vi "preview date info.vi"(6 "DateTimeOrginal":timestamp, 8 "error in":errorcluster, 11 "Cluster in":T1={"Running VI"=refnum, "Test VI"=refnum, "Q Ref"=refnum, "UE"=refnum, "Data"=variant, "Timeout"=-1, "ListBox[]"=[], "Source Path"=path "", "Delta Time"=0.0, "ExifInfo[]"=[], "ListIndex"=0, "counter"=0, "Format"=enum."Files Only", "total"=0, "Operation"=enum."Read Info", "Status"=""} {"ExifInfo[]"."New DateTime" format="%<%.3X>T"; "ExifInfo[]"."DateTimeOrginal" format="%<%.3X>T"}) -> (0 "error out":errorcluster, 3 "Cluster out":T1={"Running VI"=refnum, "Test VI"=refnum, "Q Ref"=refnum, "UE"=refnum, "Data"=variant, "Timeout"=-1, "ListBox[]"=[], "Source Path"=path "", "Delta Time"=0.0, "ExifInfo[]"=[], "ListIndex"=0, "counter"=0, "Format"=enum."Files Only", "total"=0, "Operation"=enum."Read Info", "Status"=""} {"ExifInfo[]"."New DateTime" format="%<%.3X>T"; "ExifInfo[]"."DateTimeOrginal" format="%<%.3X>T"})   [LabVIEW 2023, in "EXIF Modifier.lvlib"]
uses:
  Controls/exif_consumer cluster.ctl
  Controls/exif_info cluster.ctl
  EXIF Modifier.lvlib
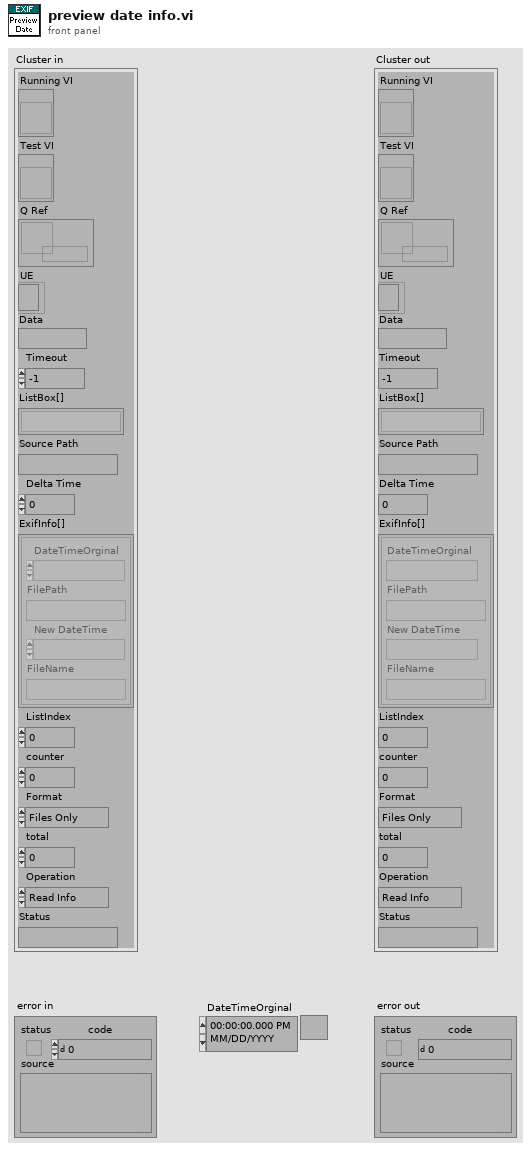
[diagram p1: front panel]
types:
  T1 = typedef "EXIF Modifier.lvlib/exif_consumer cluster.ctl" = cluster{"Running VI":refnum<vi>, "Test VI":refnum<vi>, "Q Ref":refnum<queue>, "UE":refnum<event-registration>, "Data":variant, "Timeout":i32, "ListBox[]":string[][], "Source Path":path, "Delta Time":dbl, "ExifInfo[]":T2[], "ListIndex":i32, "counter":i32, "Format":enum16{"Files Only", "Files Date", "All"}, "total":i32, "Operation":enum16{"Read Info", "Write Info"}, "Status":string}
  T2 = typedef "EXIF Modifier.lvlib/exif_info cluster.ctl" = cluster{"DateTimeOrginal":timestamp, "FilePath":path, "New DateTime":timestamp, "FileName":string}
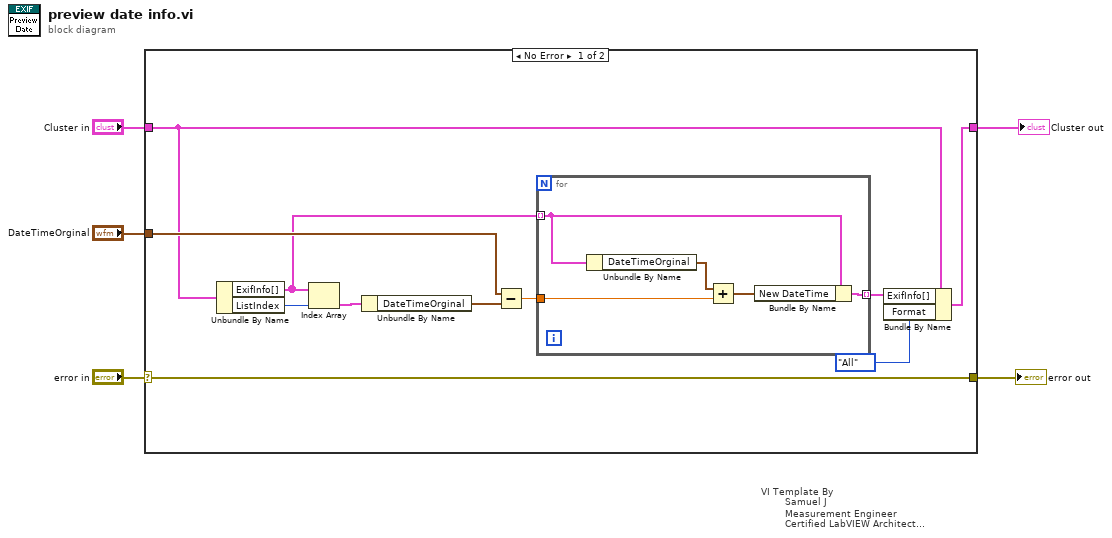
[diagram p0: block diagram]
diagram:
  n1 = case "VI Template By\n        Samuel J\n        Measurement Engineer\n        Certified LabVIEW Architect\n        Vestas Technology R&D Chennai" shown="No Error" "error in" {
    selector: "error in" -> [w16 w23]
    tunnel: [w16 w23] -> w4
    tunnel: [w7 w22] -> w2
    tunnel: "Cluster in" -> [w8 w22]
    tunnel: "DateTimeOrginal" -> [w12 _]
    frame No Error {
      n2 = Unbundle By Name(w8) -> ("ExifInfo[]"=w11:T2[], "ListIndex"=w15:i32)
      n3 = Index Array(array=w11, index=w15) -> (element=w14:T2)
      n4 = Unbundle By Name(w14) -> ("DateTimeOrginal"=w13:timestamp)
      n5 = Subtract(x=w12, y=w13) -> (x-y=w10:dbl)
      n6 = for {
        tunnel: w11 -> [w21] mode=indexing
        tunnel: w10 -> [w19]
        tunnel: [w17] -> w9 mode=indexing
        n7 = Unbundle By Name(w21) -> ("DateTimeOrginal"=w20:timestamp)
        n8 = Add(x=w20, y=w19) -> (x+y=w18:timestamp)
        n9 = Bundle By Name(cluster=w21, "New DateTime"=w18) -> (w17:T2)
      }
      n10 = Bundle By Name(cluster=w8, "ExifInfo[]"=w9, "Format"=enum16{"Files Only", "Files Date", "All"}."All") -> (w7:T1)
    }
    frame Error {
    }
  }
  "error out" <- w4
  "Cluster out" <- w2
